vi "Show Front.vi"(8 "error in (no error)":errorcluster, 11 "Abstruct View in":refnum<class "Abstruct View.lvclass">) -> (0 "error out":errorcluster, 3 "Abstruct View out":refnum<class "Abstruct View.lvclass">)   [LabVIEW 2020, in "Abstruct View.lvlib" / "Abstruct View.lvclass"]
uses:
  Abstruct View.lvclass
  Abstruct View.lvclass/Abstruct View.ctl
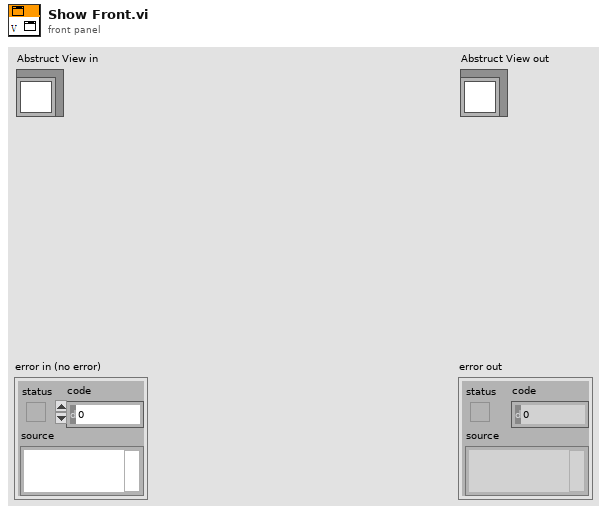
[diagram p1: front panel]
types:
  T1 = enum32{"Invalid", "Standard", "Closed", "Hidden", "Minimized", "Maximized"}
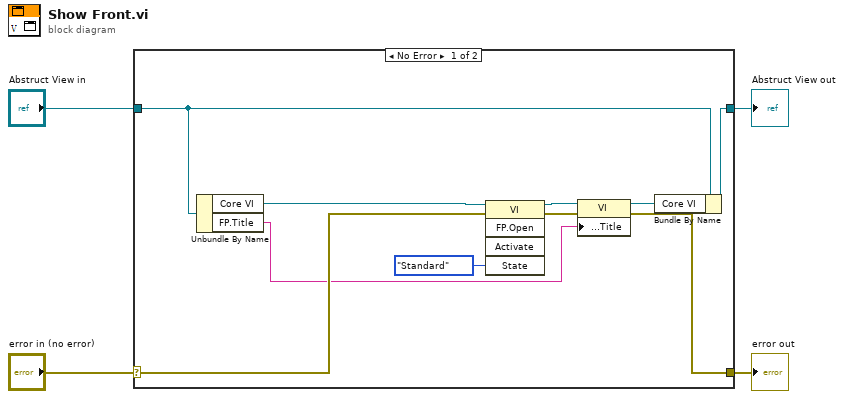
[diagram p0: block diagram]
diagram:
  n1 = case shown="No Error" "error in (no error)" {
    selector: "error in (no error)" -> [w11 w15]
    tunnel: [w7 w15] -> w3
    tunnel: [w8 w14] -> w1
    tunnel: "Abstruct View in" -> [w10 w14]
    frame No Error {
      n2 = Unbundle By Name(w10) -> ("Core VI"=w12:refnum<vi>, "FP.Title"=w5:string)
      n3 = invoke class="VI" method="FP.Open"(reference=w12, error in=w11, "State"=T1."Standard") -> (reference out=w9:refnum<vi>, error out=w7:errorcluster)  [unwired: 2 in, 3 out]
      n4 = property class="VI"(reference=w9, "Front Panel.Title"=w5) -> (reference out=w6:refnum<vi>)  [unwired: 1 in, 1 out]
      n5 = Bundle By Name(cluster=w10, "Core VI"=w6) -> (w8:refnum<class "Abstruct View.lvclass">)
    }
    frame Error {
    }
  }
  "error out" <- w3
  "Abstruct View out" <- w1
